vi "Equi-Ripple BandPass (CDB).vi"(0 "X":cdb[](array[numeric]), 1 "lower pass freq":dbl=0.25000000000000006 format="%0.2f", 3 "# of taps":i32=32, 4 "lower stop freq":dbl=0.2 format="%0.2f", 5 "higher pass freq":dbl=0.3500000000000001 format="%0.2f", 8 "higher stop freq":dbl=0.4000000000000001 format="%0.2f", 9 "sampling freq: fs":dbl=1.0 format="%0.2f") -> (6 "Filtered X":cdb[](array[numeric]), 7 "error":i32)   [LabVIEW 2020, in "NI_AALBase.lvlib"]
doc: "Generates a bandpass FIR filter with equi-ripple characteristics using the Parks-McClellan algorithm and the <B>higher pass freq</B>, <B>lower pass freq</B>, <B># of taps</B>, <B>lower stop freq</B>, <B>higher stop freq</B>, and <B>sampling freq: fs</B>. The Equi-Ripple BandPass VI then applies a linear-phase, bandpass filter to the input sequence <B>X</B> using the Convolution VI to obtain <B>Filtered X</B>. Wire data to the <B>X</B> input to determine the polymorphic instance to use or manually select the instance."
uses:
  NI_AALBase.lvlib
  1D Convolution (DBL).vi
  NI_AALPro.lvlib
panel:
  # "Equi-Ripple\n Bandpass FIR Filter"
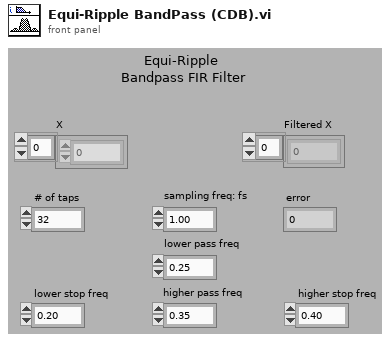
[diagram p1: front panel]
types:
  T1 = cluster{"Amplitude":dbl, "DC":dbl, "lower stop freq":dbl, "Weight":dbl}
  T2 = cluster{"Amplitude":dbl, "lower pass freq":dbl, "higher pass freq":dbl, "Weight":dbl}
  T3 = cluster{"Amplitude":dbl, "higher stop freq":dbl, dbl, "Weight":dbl}
  T4 = cluster{"Amplitude":dbl, "higher stop freq":dbl, "higher pass freq":dbl, "Weight":dbl}[]
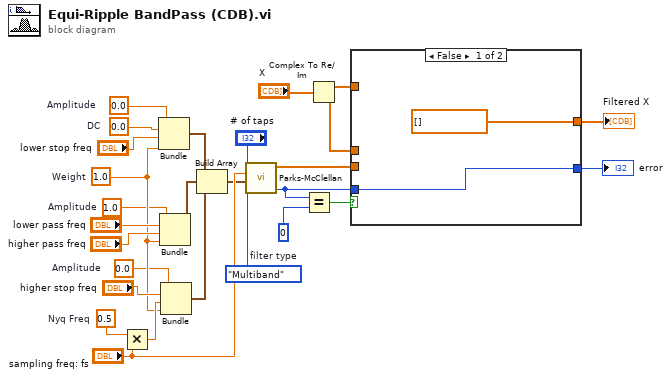
[diagram p0: block diagram]
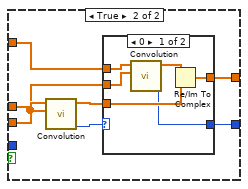
[diagram p2: hidden frame]
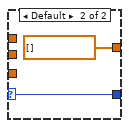
[diagram p3: hidden frame]
diagram:
  w16 = enum32{"Multiband", "Differentiator", "Hilbert"}."Multiband"  # filter type
  w10 = 0.0  # Amplitude
  w9 = 0.5  # Nyq Freq
  w11 = 1.0  # Amplitude
  w12 = 1.0  # Weight
  w13 = 0.0  # DC
  w14 = 0.0  # Amplitude
  n1 = Multiply(x=w9, y="sampling freq: fs") -> (x*y=w20:dbl)
  n2 = Bundle("Amplitude"=w14, "DC"=w13, "lower stop freq"="lower stop freq", "Weight"=w12) -> (w25:T1)  [unwired: 1 in]
  n3 = Bundle("Amplitude"=w11, "lower pass freq"="lower pass freq", "higher pass freq"="higher pass freq", "Weight"=w12) -> (w24:T2)  [unwired: 1 in]
  n4 = Bundle("Amplitude"=w10, "higher stop freq"="higher stop freq", w20, "Weight"=w12) -> (w19:T3)  [unwired: 1 in]
  n5 = Build Array(w25, w24, w19) -> (w17:T4)
  n6 = call "Parks-McClellan.vi"("filter type"=w16, "Band Parameters"=w17, "sampling freq: fs"="sampling freq: fs", "# of taps"="# of taps") -> ("error"=w7:i32, "h"=w6:dbl[])  [unwired: 1 out]
  n7 = Equal?(x=w7, y=0) -> (x = y?=w8:bool)
  n8 = Complex To Re/Im(x + iy="X") -> (x=w4:dbl[], y=w3:dbl[])
  n9 = case shown="False" w8 {
    tunnel: w7 -> [w29 _]
    tunnel: [w29 w30] -> w1
    tunnel: [cdb[] [] ("empty array") w32] -> w2
    tunnel: w3 -> [_ w36]
    tunnel: w6 -> [_ w33]
    tunnel: w4 -> [_ w34]
    frame False {
    }
    frame True {
      n10 = call-poly "Convolution.vi"("Y"=w33, "X"=w36) -> ("error"=w35:i32, "X * Y"=w31:dbl[])  [unwired: 8 in]
      n11 = case shown="0" w35 {
        selector: w35 -> [_ w43]
        tunnel: w34 -> [w42 _]
        tunnel: w33 -> [w41 _]
        tunnel: [w39 cdb[] [] ("empty array")] -> w32
        tunnel: w31 -> [w40 _]
        tunnel: [w38 w43] -> w30
        frame 0 {
          n12 = call-poly "Convolution.vi"("Y"=w41, "X"=w42) -> ("error"=w38:i32, "X * Y"=w37:dbl[])  [unwired: 8 in]
          n13 = Re/Im To Complex(1:w40, 2:w37) -> (0:w39:cdb[])
        }
        frame Default {
        }
      }
    }
  }
  "Filtered X" <- w2
  "error" <- w1
